vi "WriteArrayAsImage.vi"(9 "Data":sgl[][](graph), 10 "File Path":path, 11 "Normalize Mode":T1(ring)) -> ()   [LabVIEW 2011]
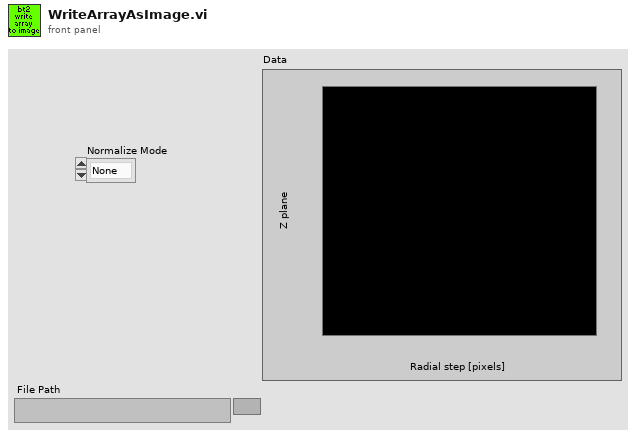
[diagram p1: front panel]
types:
  T1 = enum16{"None", "Normalize", "NormalizeWithoutOffset"}
  T2 = typedef "IMAQ Image.ctl" = refnum<image>
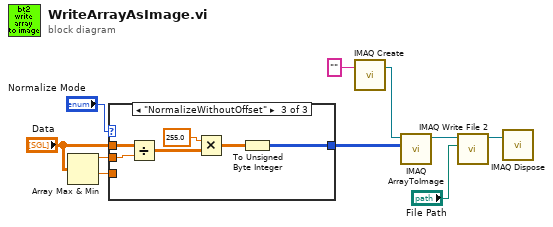
[diagram p0: block diagram]
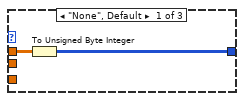
[diagram p2: hidden frame]
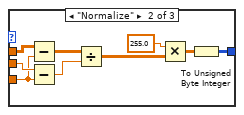
[diagram p3: hidden frame]
diagram:
  n1 = Array Max & Min(array="Data") -> (max value=w2:sgl, min value=w3:sgl)  [unwired: 2 out]
  n2 = case shown="\"NormalizeWithoutOffset\"" "Normalize Mode" {
    tunnel: [w12 w13 w23] -> w5
    tunnel: "Data" -> [w11 w21 w26]
    tunnel: w3 -> [_ w18 _]
    tunnel: w2 -> [_ w19 w27]
    frame "None", Default {
      n3 = To Unsigned Byte Integer(number=w11) -> (unsigned 8bit integer=w12:u8[][])
    }
    frame "Normalize" {
      n4 = Subtract(x=w21, y=w18) -> (x-y=w20:sgl[][])
      n5 = Subtract(x=w19, y=w18) -> (x-y=w17:sgl)
      n6 = Divide(x=w20, y=w17) -> (x/y=w16:sgl[][])
      n7 = Multiply(x=sgl 255.0, y=w16) -> (x*y=w14:sgl[][])
      n8 = To Unsigned Byte Integer(number=w14) -> (unsigned 8bit integer=w13:u8[][])
    }
    frame "NormalizeWithoutOffset" {
      n9 = Divide(x=w26, y=w27) -> (x/y=w24:sgl[][])
      n10 = Multiply(x=sgl 255.0, y=w24) -> (x*y=w22:sgl[][])
      n11 = To Unsigned Byte Integer(number=w22) -> (unsigned 8bit integer=w23:u8[][])
    }
  }
  n12 = call "IMAQ Create"("Image Name"="") -> ("New Image"=w10:T2)  [unwired: 4 in, 1 out]
  n13 = call "IMAQ ArrayToImage"("Image Pixels (U8)"=w5, "Image"=w10) -> ("Image Out"=w8:T2)  [unwired: 8 in, 1 out]
  n14 = call-poly "IMAQ Write File 2"("File Path"="File Path", "Image"=w8) -> ("Image Out (duplicate)"=w7:T2)  [unwired: 8 in, 1 out]
  n15 = call "IMAQ Dispose"("Image"=w7) -> ()  [unwired: 5 in, 1 out]
